vi "Current VIs Parent Directory__ogtk.vi"(4 "Relative path (.)":path=path "") -> (1 "Parent Directory (+ Relative)":path)   [LabVIEW 2009]
doc: "Gets the path to the parent directory of the calling VI. This may be used for building a path to a config file that exists in that directory or a directory relative to it. This function will move up the file structure until it reaches and Operating System Directory. It will not return the path to a built EXE or to an LLB."
uses:
  Strip Path - Traditional__ogtk.vi
panel:
  # "Current VI's Parent Directory.vi\n\nGets the path to the parent directory of the calling VI.\n\nPlease visit http://www.OpenG.org to learn about the\nOpen Source LabVIEW software movement.\n\nNOTICE -- YOU MUST LEAVE THIS NOTICE IN PLACE.  PER THE TERMS OF THE LICENSE BELOW, YOU MAY SUBLICENSE THIS SOFTWARE \nIN ANY WAY THAT DOES NOT CONFLICT WITH THIS LICENSE.\n\n### BSD License (http://www.opensource.org/licenses/bsd-license.php) Begin ###\n \nCopyright (c) 2002, Jim Kring <jim@jimkring.com>\nCopyright (c) 2002, Cal-Bay Systems, Inc. <info@calbay.com>\n\nAll rights reserved.\n\nRedistribution and use in source and binary forms, with or without modification, are permitted provided that the following conditions are met:\n\n    * Redistributions of source code must retain the above copyright notice, this list of conditions and the following disclaimer.\n    * Redistributions in binary form must reproduce the above copyright notice, this list of conditions and the following disclaimer in the \n       documentation and/or other materials provided with the distribution.\n    * Neither the name of SciWare, James Kring, Inc., nor the names of its contributors may be used to endorse or promote products derived \n       from this software without specific prior written permission.\n\nTHIS SOFTWARE IS PROVIDED BY THE COPYRIGHT HOLDERS AND CONTRIBUTORS \"AS IS\" AND ANY EXPRESS OR IMPLIED WARRANTIES, \nINCLUDING, BUT NOT LIMITED TO, THE IMPLIED WARRANTIES OF MERCHANTABILITY AND FITNESS FOR A PARTICULAR PURPOSE ARE \nDISCLAIMED. IN NO EVENT SHALL THE COPYRIGHT OWNER OR CONTRIBUTORS BE LIABLE FOR ANY DIRECT, INDIRECT, INCIDENTAL,\n SPECIAL, EXEMPLARY, OR CONSEQUENTIAL DAMAGES (INCLUDING, BUT NOT LIMITED TO, PROCUREMENT OF SUBSTITUTE GOODS OR \nSERVICES; LOSS OF USE, DATA, OR PROFITS; OR BUSINESS INTERRUPTION) HOWEVER CAUSED AND ON ANY THEORY OF LIABILITY, \nWHETHER IN CONTRACT, STRICT LIABILITY, OR TORT (INCLUDING NEGLIGENCE OR OTHERWISE) ARISING IN ANY WAY OUT OF THE USE \nOF THIS SOFTWARE, EVEN IF ADVISED OF THE POSSIBILITY OF SUCH DAMAGE.\n\n### BSD License End ###"
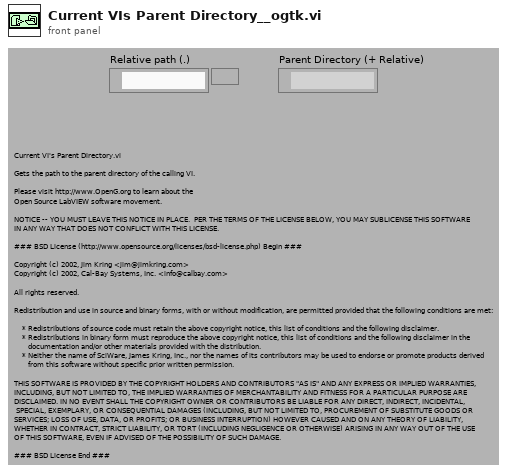
[diagram p1: front panel]
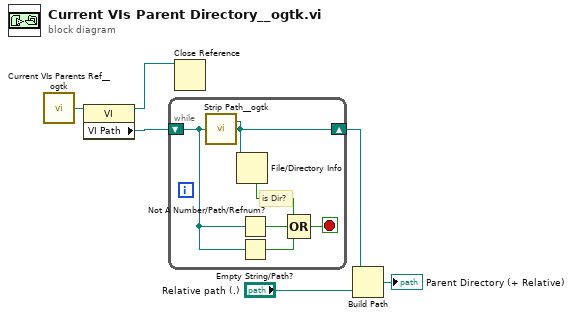
[diagram p0: block diagram]
diagram:
  n1 = call <userlib>:"Current VIs Parents Ref__ogtk.vi"() -> ("Calling VI's reference"=w6:refnum<vi>)  [unwired: 2 in]
  n2 = property class="VI"(reference=w6) -> (reference out=w4:refnum<vi>, "VI Path"=w5:path)  [unwired: 1 in, 1 out]
  n3 = while {
    shift-right: [w7] -> w1
    shift-left: w5 -> [w9]
    stop <- w11 stop-if-true
    # "is Dir?"
    n4 = call-poly "Strip Path__ogtk.vi"("path"=w9) -> ("stripped path"=w7:path)  [unwired: 1 out]
    n5 = File/Directory Info(path=w7) -> (directory=w12:bool)  [unwired: 1 in, 6 out]
    n6 = Not A Number/Path/Refnum?(number/path/refnum=w9) -> (NaN/Path/Refnum?=w10:bool)
    n7 = Empty String/Path?(string/path=w9) -> (empty?=w8:bool)
    n8 = Compound Arithmetic op=OR(w12, w10, w8) -> (w11:bool)
  }
  n9 = Close Reference(reference=w4) -> ()  [unwired: 1 in, 1 out]
  n10 = Build Path(base path=w1, name or relative path="Relative path (.)") -> (appended path=→"Parent Directory (+ Relative)":path)
